vi "nanocal -- nuclear schottky fit V5.vi"() -> ()   [LabVIEW 2020] (continued)
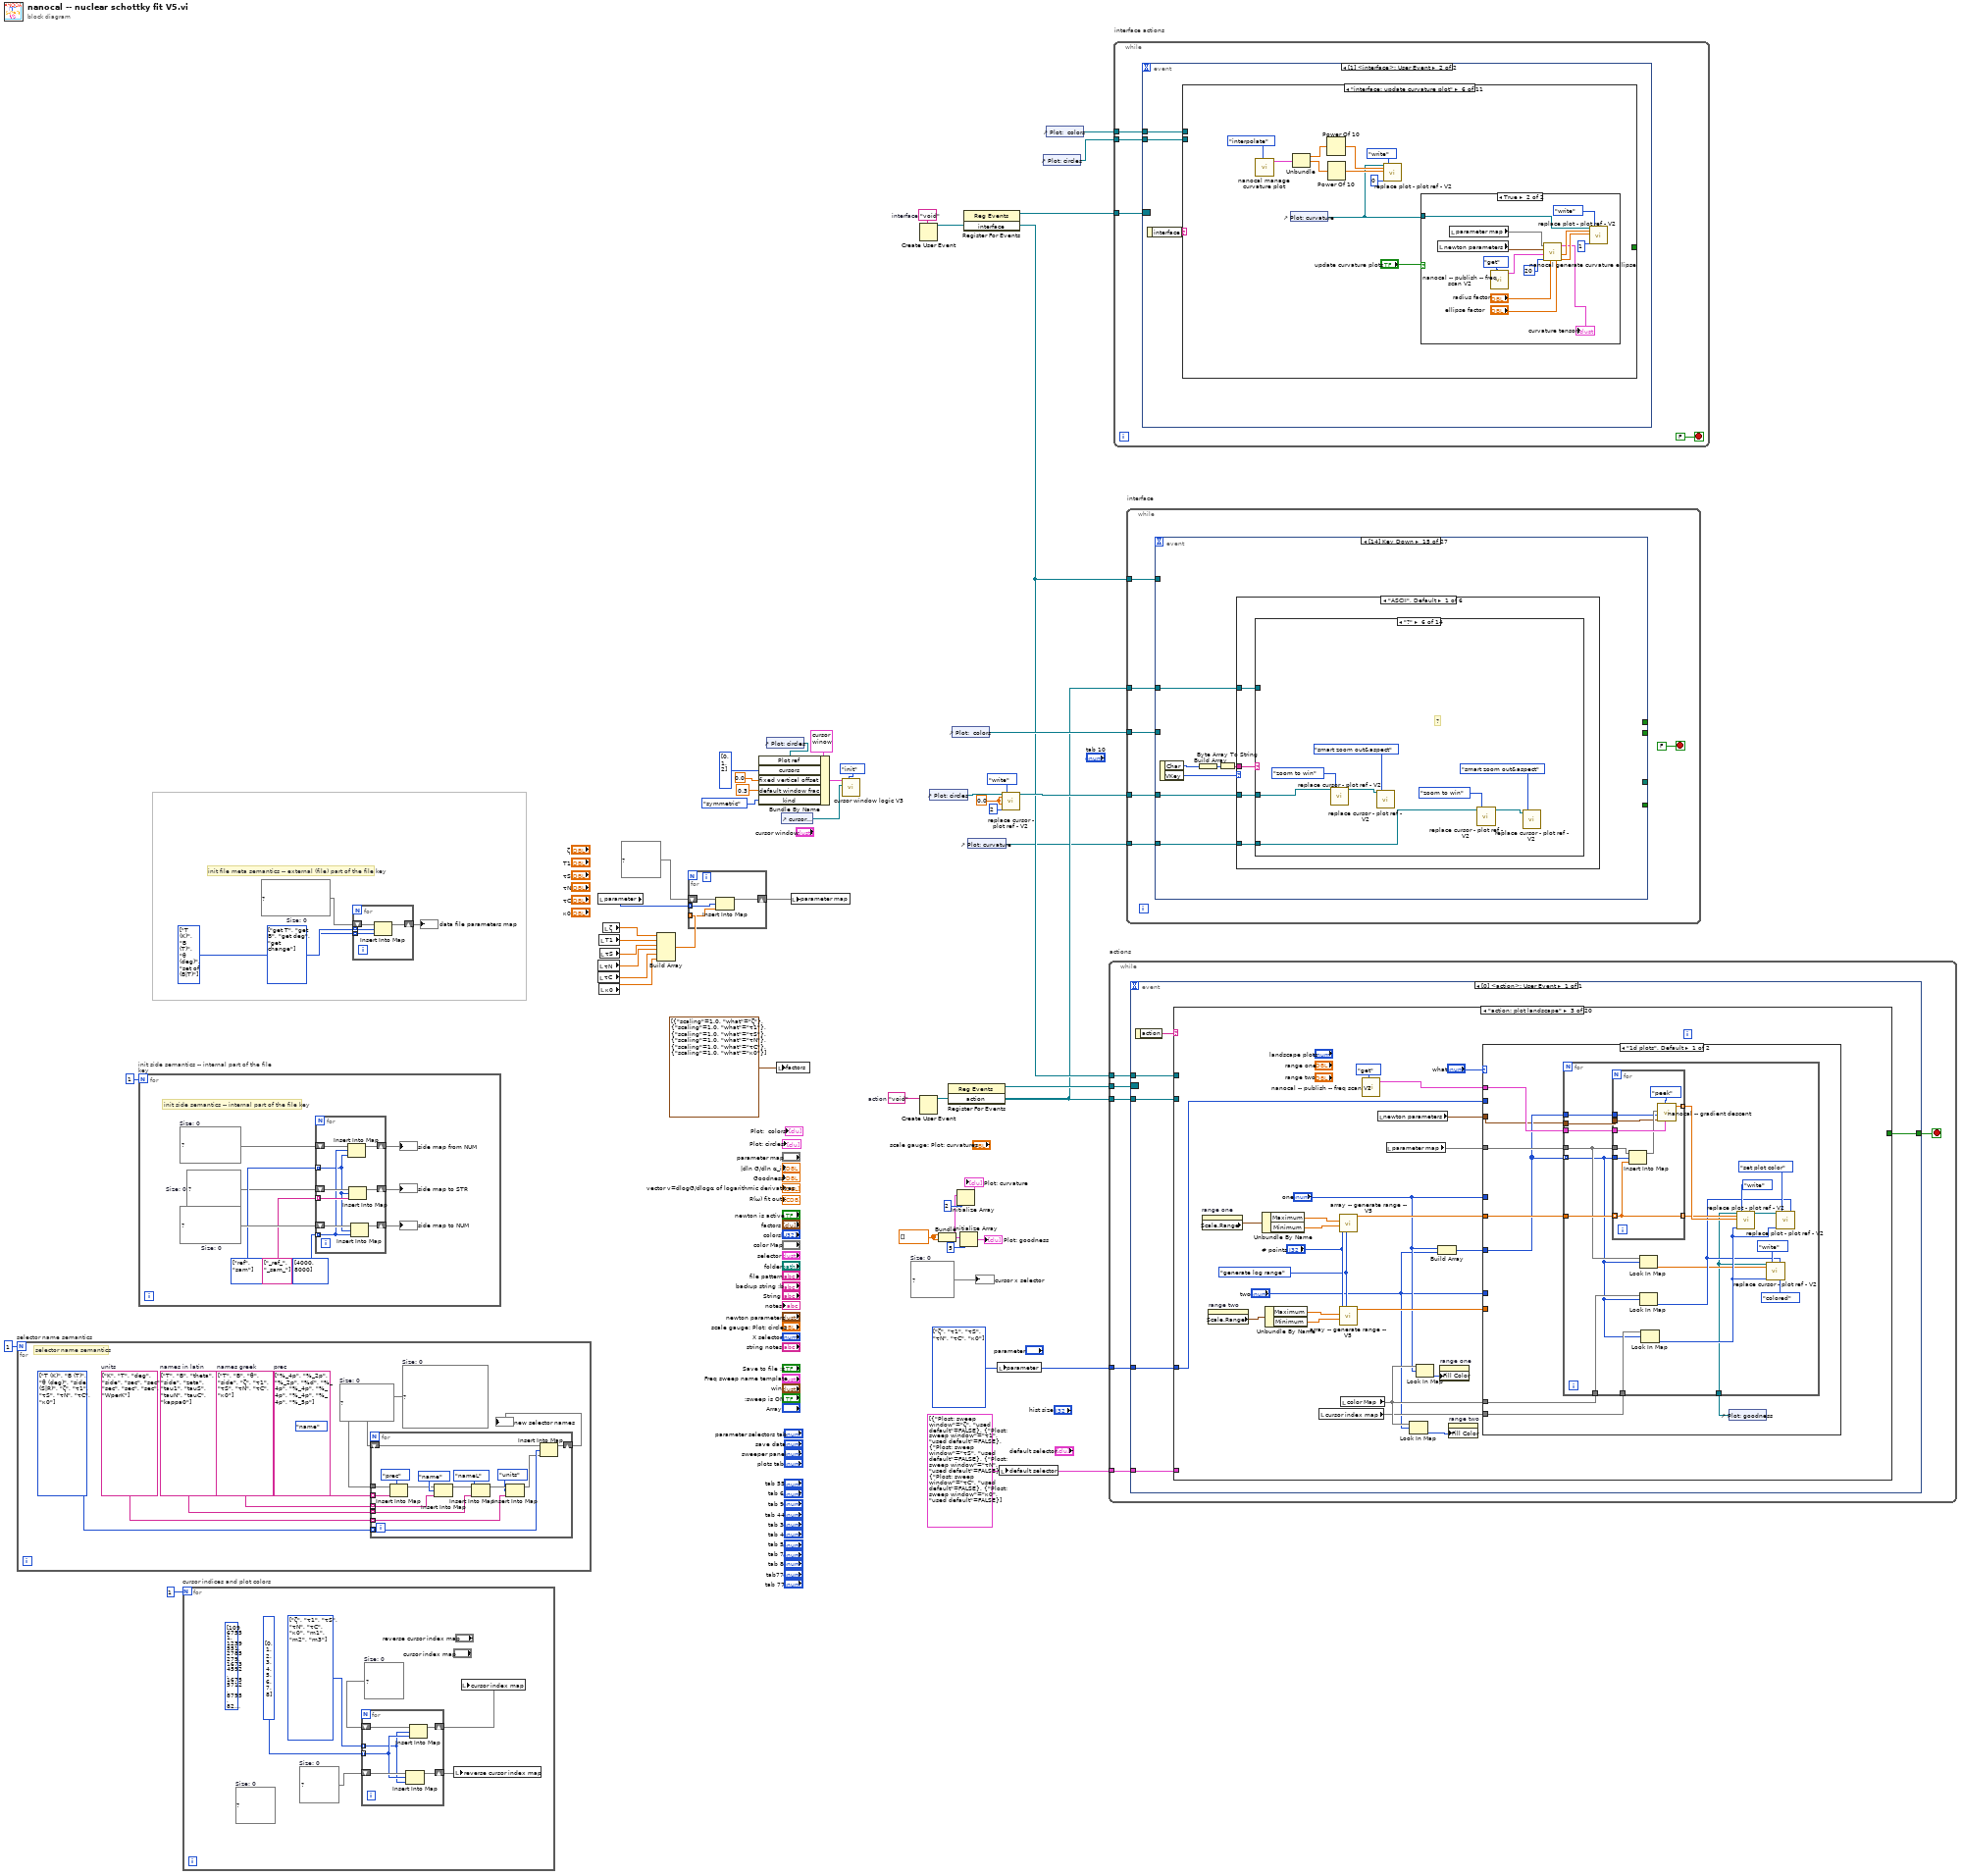
[diagram p0: block diagram]
diagram:
  w24 = T14 [{"Plost: sweep window"=enum."ζ", "used default"=FALSE}, {"Plost: sweep window"=enum."τ1", "used default"=FALSE}, {"Plost: sweep window"=enum."τS", "used default"=FALSE}, {"Plost: sweep window"=enum."τN", "used default"=FALSE}, {"Plost: sweep window"=enum."τC", "used default"=FALSE}, {"Plost: sweep window"=enum."κ0", "used default"=FALSE}] ("parameter 2")
  w25 = T12[] [enum."get T", enum."get B", enum."get deg", enum."get change"] items=["rewrite", "parse", "force pattern", "uniquenum", "get T", "get B", "get ind", "get deg", "get name", "get folder", "get extension", "get basename", "get side", "get change", "getID", "getIDStock"]
  w27 = map{T4, T12} {}  # Size: 0
  w26 = T4[] [enum."T (K)", enum."B (T)", enum."θ (deg)", enum."set of (B|T)"] items=["ζ", "τ1", "τS", "τN", "τC", "κ0", "m1", "m2", "m3", "T (K)", "B (T)", "θ (deg)", "side (S|R)", "set of (B|T)", "Re(offset)", "Im(offset)"]
  w31 = dbl[] []
  w20 = T4[] [enum."ζ", enum."τ1", enum."τS", enum."τN", enum."τC", enum."κ0"] items=["ζ", "τ1", "τS", "τN", "τC", "κ0", "m1", "m2", "m3", "T (K)", "B (T)", "θ (deg)", "side (S|R)", "set of (B|T)", "Re(offset)", "Im(offset)"]
  w34 = map{T4, dbl} {}  # Size: 0
  w35 = 0.0 ("new X")
  w48 = "void"  # interface
  w49 = "void"  # action
  # "init file meta semantics -- external (file) part of the file key"
  n1 = for "selector name semantics" {
    N: 1 -> [_]
    w51 = string[] ["%_4p", "%_2p", "%_2p", "%d", "%_4p", "%_4p", "%_4p", "%_4p", "%_4p", "%_5p"]  # prec
    w55 = map{T13, string} {}  # Size: 0
    (unwired) nameformattingitem."name" ("name formatting item")
    w53 = string[] ["K", "T", "deg", "side", "sec", "sec", "sec", "sec", "sec", "WperK"]  # units
    w56 = string[] ["T", "B", "theta", "side", "zeta", "tau1", "tauS", "tauN", "tauC", "kappa0"]  # names in latin
    w54 = string[] ["T", "B", "θ", "side", "ζ", "τ1", "τS", "τN", "τC", "κ0"]  # names greek
    w58 = map{T4, map{T13, string}} {}  # Size: 0
    w57 = T4[] [enum."T (K)", enum."B (T)", enum."θ (deg)", enum."side (S|R)", enum."ζ", enum."τ1", enum."τS", enum."τN", enum."τC", enum."κ0"] items=["ζ", "τ1", "τS", "τN", "τC", "κ0", "m1", "m2", "m3", "T (K)", "B (T)", "θ (deg)", "side (S|R)", "set of (B|T)", "Re(offset)", "Im(offset)"]
    # "selector name semantics"
    n2 = for {
      shift-right: [w73] -> w52
      shift-left: w58 -> [w74]
      tunnel: w56 -> [w64] mode=indexing
      tunnel: w57 -> [w72] mode=indexing
      tunnel: w55 -> [w62]
      tunnel: w54 -> [w63] mode=indexing
      tunnel: w53 -> [w65] mode=indexing
      tunnel: w51 -> [w61] mode=indexing
      n3 = Insert Into Map(map in=w62, key=nameformattingitem."prec", value=w61) -> (map out=w60:map{T13, string})  [unwired: 2 out]
      n4 = Insert Into Map(map in=w60, key=nameformattingitem."name", value=w63) -> (map out=w71:map{T13, string})  [unwired: 2 out]
      n5 = Insert Into Map(map in=w71, key=nameformattingitem."nameL" ("name formatting item"), value=w64) -> (map out=w70:map{T13, string})  [unwired: 2 out]
      n6 = Insert Into Map(map in=w70, key=nameformattingitem."units" ("name formatting item"), value=w65) -> (map out=w69:map{T13, string})  [unwired: 2 out]
      n7 = Insert Into Map(map in=w74, key=w72, value=w69) -> (map out=w73:map{T4, map{T13, string}})  [unwired: 2 out]
    }
    "new selector names" <- w52
  }
  n8 = for "init side semantics -- internal part of the file key" {
    N: 1 -> [_]
    w76 = map{i32, T11} {}  # Size: 0
    w78 = map{T11, string} {}  # Size: 0
    w79 = T11[] [enum."ref", enum."sam"] items=["sam", "ref"]
    w83 = map{T11, i32} {}  # Size: 0
    # "init side semantics -- internal part of the file key"
    n9 = for {
      shift-right: [w91] -> w80
      shift-left: w83 -> [w92]
      tunnel: string[] ["_ref_", "_sam_"] -> [w88] mode=indexing
      tunnel: i32[] [4000, 8000] -> [w85] mode=indexing
      tunnel: w79 -> [w84] mode=indexing
      shift-right: [w89] -> w77
      shift-left: w78 -> [w90]
      shift-right: [w86] -> w75
      shift-left: w76 -> [w87]
      n10 = Insert Into Map(map in=w87, key=w85, value=w84) -> (map out=w86:map{i32, T11})  [unwired: 2 out]
      n11 = Insert Into Map(map in=w90, key=w84, value=w88) -> (map out=w89:map{T11, string})  [unwired: 2 out]
      n12 = Insert Into Map(map in=w92, key=w84, value=w85) -> (map out=w91:map{T11, i32})  [unwired: 2 out]
    }
    "side map from NUM" <- w75
    "side map to STR" <- w77
    "side map to NUM" <- w80
  }
  n13 = for "cursor indices and plot colors" {
    N: 1 -> [_]
    (unwired) map{T4, i32} {}  # Size: 0
    w94 = map{i32, T4} {}  # Size: 0
    (unwired) u32[] [10967551, 1239551, 2785279, 16734592, 16755712, 8795, 8285330, 9272482, 9204890]
    w98 = map{T4, i32} {}  # Size: 0
    w95 = T4[] [enum."ζ", enum."τ1", enum."τS", enum."τN", enum."τC", enum."κ0", enum."m1", enum."m2", enum."m3"] items=["ζ", "τ1", "τS", "τN", "τC", "κ0", "m1", "m2", "m3", "T (K)", "B (T)", "θ (deg)", "side (S|R)", "set of (B|T)", "Re(offset)", "Im(offset)"]
    n14 = for {
      shift-right: [w103] -> w96
      shift-left: w98 -> [w104]
      tunnel: w95 -> [w99] mode=indexing
      tunnel: i32[] [0, 1, 2, 3, 4, 5, 6, 7, 8] -> [w100] mode=indexing
      shift-right: [w101] -> w93
      shift-left: w94 -> [w102]
      n15 = Insert Into Map(map in=w102, key=w100, value=w99) -> (map out=w101:map{i32, T4})  [unwired: 2 out]
      n16 = Insert Into Map(map in=w104, key=w99, value=w100) -> (map out=w103:map{T4, i32})  [unwired: 2 out]
    }
    n17 = local write "reverse cursor index map"(w93) -> ()
    n18 = local write "cursor index map"(w96) -> ()
  }
  n19 = for {
    shift-right: [w107] -> w28
    shift-left: w27 -> [w108]
    tunnel: w26 -> [w106] mode=indexing
    tunnel: w25 -> [w105] mode=indexing
    n20 = Insert Into Map(map in=w108, key=w106, value=w105) -> (map out=w107:map{T4, T12})  [unwired: 2 out]
  }
  "data file parameters map" <- w28
  n21 = local read "parameter"() -> (w18:T4[])
  n22 = local read "τN"() -> (w14:dbl)
  n23 = local read "τC"() -> (w15:dbl)
  n24 = local read "T1"() -> (w12:dbl)
  n25 = local read "κ0"() -> (w16:dbl)
  n26 = local read "τS"() -> (w13:dbl)
  n27 = local read "ζ"() -> (w11:dbl)
  n28 = Build Array(w11, w12, w13, w14, w15, w16) -> (w17:dbl[])
  n29 = for {
    shift-right: [w111] -> w19
    shift-left: map{T4, dbl} {} ("Map IN") -> [w112]
    tunnel: w18 -> [w110] mode=indexing
    tunnel: w17 -> [w109] mode=indexing
    n30 = Insert Into Map(map in=w112, key=w110, value=w109) -> (map out=w111:map{T4, dbl})  [unwired: 2 out]
  }
  n31 = control-ref of="Plot: circles"() -> (w40:refnum<vi>)
  n32 = Bundle By Name(cluster=T17 {"left"=0.0, "right "=0.0, "center"=0.0, "window"=0.0, "cursors"=[], "relative"=0, "absolute"=0, "fixed vertical offset"=0.0, "vertical offset"=0.0, "skew"=0.0, "default window frac"=0.0, "kind"=enum."symmetric", "skew.left"=0.0, "skew.right"=0.0, "Plot ref"=refnum, "wing order"=enum."forw"} ("cursor bracket: All, data window"), "Plot ref"=w40, "cursors"=i32[] [0, 1, 2], "fixed vertical offset"=0.0, "default window frac"=0.3 ("fixed vertical offset"), "kind"=enum16{"symmetric", "skewed", "fancy"}."symmetric") -> (w43:T17)
  n33 = local write "factors"(cluster{"scaling":dbl, "what":T4}[] [{"scaling"=1.0, "what"=enum."ζ"}, {"scaling"=1.0, "what"=enum."τ1"}, {"scaling"=1.0, "what"=enum."τS"}, {"scaling"=1.0, "what"=enum."τN"}, {"scaling"=1.0, "what"=enum."τC"}, {"scaling"=1.0, "what"=enum."κ0"}]) -> ()
  n34 = control-ref of="cursor window"() -> (w39:refnum<vi>)
  n35 = local write "parameter map"(w19) -> ()
  n36 = call "cursor window logic V3.vi"("cursor window action"=cursor_window_action."init", "cursor window in"=w39, "cursor window init"=w43) -> ()  [unwired: 7 in, 2 out]
  n37 = Create User Event(user event datatype=w48) -> (user event=w8:refnum<user-event>)  [unwired: 1 in, 1 out]
  n38 = Create User Event(user event datatype=w49) -> (user event=w7:refnum<user-event>)  [unwired: 1 in, 1 out]
  n39 = control-ref of="Plot: circles"() -> (w36:refnum<vi>)
  n40 = Bundle(w31, w31) -> (w3:cluster{dbl[], dbl[]})  [unwired: 1 in]
  n41 = register-events(w7) -> (reference out=w50:refnum<event-registration>)  [unwired: 2 in, 1 out]
  n42 = control-ref of="Plot:  colors"() -> (w33:refnum<vi>)
  n43 = Initialize Array(w3, 2 ("dimension size")) -> (→"Plot: curvature":cluster{dbl[], dbl[]}[])
  n44 = Initialize Array(w3, 5 ("dimension size")) -> (→"Plot: goodness":cluster{dbl[], dbl[]}[])
  n45 = register-events(w8) -> (reference out=w9:refnum<event-registration>)  [unwired: 2 in, 1 out]
  n46 = control-ref of="Plot: curvature"() -> (w1:refnum<vi>)
  n47 = local write "parameter"(w20) -> ()
  n48 = local write "default selector"(w24) -> ()
  n49 = call "replace cursor - plot ref - V2.vi"("Plot ref in"=w36, "new X"=w35, "new  Y"=w35, "cursor index"=2, "cursor action"=cursor_action."write") -> ()  [unwired: 11 in, 4 out]
  n50 = control-ref of="Plot: circles"() -> (w5:refnum<vi>)
  n51 = control-ref of="Plot:  colors"() -> (w6:refnum<vi>)
  n52 = while "actions" {
    tunnel: w50 -> [w118]
    tunnel: w7 -> [w117]
    tunnel: w8 -> [w115]
    tunnel: w20 -> [w114]
    tunnel: w24 -> [w113]
    stop <- w116 stop-if-true
    n53 = event shown="[0] <action>: User Event" {
      selector: w118 -> [_]
      dyn-events: _ -> [_]
      timeout: _ -> [_]
      tunnel: w117 -> [w123]
      tunnel: [w122] -> w116
      tunnel: w115 -> [w121]
      tunnel: w114 -> [w120]
      tunnel: w113 -> [w119]
      event User Event {
        n54 = event-data() -> ("action"=w124:string)  [unwired: 1 in]
        n55 = case shown="\"action: plot landscape\"" w124 {
          tunnel: w123 -> [w132 _ _ _ w328 w353 _ _ w546 _ w673 _ _ w777 w829 w910 _ w968 _ _]
          tunnel: [_ _ _ _ _ _ _ _ _ _ _ _ _ _ _ _ TRUE _ _ _] -> w122
          tunnel: w121 -> [w135 w139 _ w263 w322 _ _ _ _ _ _ _ w686 _ w819 _ _ _ _ _]
          tunnel: w120 -> [_ w146 w155 w262 _ _ w480 _ _ _ _ _ w687 _ w825 _ _ _ _ _]
          tunnel: w119 -> [_ _ _ _ _ _ _ _ _ _ _ _ _ _ _ _ _ _ _ _]
          frame "action: new sweep" {
            n56 = Generate User Event(user event=w135, event data cluster="interface: update plot colors cursors" ("event data")) -> (user event out=w136:refnum<user-event>)  [unwired: 2 in, 1 out]
            n57 = Generate User Event(user event=w136, event data cluster="interface: reset colors" ("event data")) -> ()  [unwired: 2 in, 2 out]
            n58 = Generate User Event(user event=w132, event data cluster="action: replot circles" ("event data")) -> ()  [unwired: 2 in, 2 out]
            n59 = call "nanocal -- publish -- freq scan V2.vi"("publisher action"=publisher_action."get") -> ("z out (V)"=w131:cdb[])  [unwired: 7 in, 3 out]
            n60 = control-ref of="Plot: circles"() -> (w126:refnum<vi>)
            n61 = Complex To Re/Im(x + iy=w131) -> (x=w129:dbl[], y=w130:dbl[])
            n62 = call "replace plot - plot ref - V2.vi"("Plot ref in"=w126, "Array X IN"=w129, "Array Y IN"=w130, "plot index"=enum16{"data R(ω)", "fit R(ω)"}."data R(ω)" ("Plost: sweep window"), "cursor action"=cursor_action."write") -> ()  [unwired: 11 in, 4 out]
          }
          frame "action: replot circles" {
            n63 = local read "newton parameters"() -> (w147:T5)
            n64 = local read "parameter map"() -> (w141:map{T4, dbl})
            n65 = call "nanocal -- publish -- freq scan V2.vi"("publisher action"=publisher_action."get") -> ("data"=w145:T32)  [unwired: 7 in, 3 out]
            n66 = call "nanocal -- gradient descent.vi"("data"=w145, "action"=nanocal_--_gradient_descent_--_action."peek", "newton pars"=w147, "parameter keys IN"=w146, "parameter Map IN"=w141) -> ("logarithmic derivatives OUT"=w142:dbl[], "R(ω) out"=w140:cdb[], "goodness OUT"=w144:dbl)  [unwired: 2 in, 2 out]
            n67 = flat-sequence {
              tunnel: w140 -> [w150]
              tunnel: w139 -> [w152]
              tunnel: "interface: update circle fit plot" ("event data") -> [w151]
              frame #0 {
                n68 = local write "R(ω) fit out"(w150) -> ()
              }
              frame #1 {
                n69 = Generate User Event(user event=w152, event data cluster=w151) -> ()  [unwired: 2 in, 2 out]
              }
            }
            n70 = local write "Goodness"(w144) -> ()
            n71 = Absolute Value(x=w142) -> (abs(x)=w143:dbl[])
            n72 = local write "|v_i| = | dlogG/dlogα_i | (log scale slider)"(w143) -> ()
            n73 = local write "vector v=dlogG/dlogα of logarithmic derivatives"(w142) -> ()
          }
          frame "action: plot landscape" {
            w166 = array_action."generate log range" ("action")
            n74 = property on="range one" class="Slide (strict)"() -> ("Scale.Range"=w175:T34)  [unwired: 2 in, 2 out]
            n75 = property on="range two" class="Slide (strict)"() -> ("Scale.Range"=w174:T34)  [unwired: 2 in, 2 out]
            n76 = Unbundle By Name(w175) -> ("Maximum"=w169:dbl, "Minimum"=w168:dbl)
            n77 = Unbundle By Name(w174) -> ("Maximum"=w171:dbl, "Minimum"=w170:dbl)
            n78 = local read "cursor index map"() -> (w161:map{T4, i32})
            n79 = call "array -- generate range -- V5.vi"("action"=w166, "ω points"="# points", "ω from"=w168, "ω to"=w169) -> ("ω out"=w167:dbl[])  [unwired: 7 in]
            n80 = call "array -- generate range -- V5.vi"("action"=w166, "ω points"="# points", "ω from"=w170, "ω to"=w171) -> ("ω out"=w172:dbl[])  [unwired: 7 in]
            n81 = local read "color Map"() -> (w162:map{T4, u32})
            n82 = call "nanocal -- publish -- freq scan V2.vi"("publisher action"=publisher_action."get") -> ("data"=w154:T32)  [unwired: 7 in, 3 out]
            n83 = local read "newton parameters"() -> (w156:T5)
            n84 = local read "parameter map"() -> (w153:map{T4, dbl})
            n85 = Look In Map(map=w162, key="two") -> (value=w164:u32)  [unwired: 1 in, 1 out]
            n86 = Look In Map(map=w162, key="one") -> (value=w163:u32)  [unwired: 1 in, 1 out]
            n87 = Build Array("one", "two") -> (w160:T4[])
            n88 = property on="range one" class="Slide (strict)"("Fill Color"=w163) -> ()  [unwired: 2 in, 2 out]
            n89 = property on="range two" class="Slide (strict)"("Fill Color"=w164) -> ()  [unwired: 2 in, 2 out]
            n90 = case shown="\"1d plots\", Default" "what" {
              tunnel: w153 -> [w183 w223]
              tunnel: "one" -> [_ w222]
              tunnel: w172 -> [_ w221]
              tunnel: w167 -> [w182 w220]
              tunnel: "two" -> [_ w219]
              tunnel: w162 -> [w181 _]
              tunnel: w161 -> [w180 _]
              tunnel: w160 -> [w177 _]
              tunnel: w154 -> [w178 w214]
              tunnel: w156 -> [w176 w212]
              tunnel: w155 -> [_ w213]
              frame "1d plots", Default {
                n91 = control-ref of="Plot: goodness"() -> (w179:refnum<vi>)
                n92 = for {
                  tunnel: w183 -> [w190]
                  tunnel: w182 -> [w199]
                  tunnel: w177 -> [w189] mode=indexing
                  tunnel: w181 -> [w196]
                  tunnel: w180 -> [w195]
                  tunnel: w179 -> [w187]
                  tunnel: w178 -> [w186]
                  tunnel: w177 -> [w185]
                  tunnel: w176 -> [w184]
                  n93 = for {
                    tunnel: w199 -> [w203] mode=indexing
                    tunnel: [w204] -> w201 mode=indexing
                    tunnel: [w203] -> w200 mode=indexing
                    tunnel: w190 -> [w210]
                    tunnel: w189 -> [w211]
                    tunnel: w186 -> [w209]
                    tunnel: w185 -> [w206]
                    tunnel: w184 -> [w205]
                    n94 = Insert Into Map(map in=w210, key=w211, value=w203) -> (map out=w208:map{T4, dbl})  [unwired: 2 out]
                    n95 = call "nanocal -- gradient descent.vi"("data"=w209, "action"=nanocal_--_gradient_descent_--_action."peek", "newton pars"=w205, "parameter keys IN"=w206, "parameter Map IN"=w208) -> ("goodness OUT"=w204:dbl)  [unwired: 2 in, 4 out]
                  }
                  n96 = Look In Map(map=w190, key=w189) -> (value=w188:dbl)  [unwired: 1 in, 1 out]
                  n97 = Look In Map(map=w196, key=w189) -> (value=w191:u32)  [unwired: 1 in, 1 out]
                  n98 = Look In Map(map=w195, key=w189) -> (value=w193:i32)  [unwired: 1 in, 1 out]
                  n99 = call "replace plot - plot ref - V2.vi"("Plot ref in"=w187, "Array X IN"=w200, "Array Y IN"=w201, "plot index"=w193, "cursor action"=cursor_action."write") -> ("Plot ref out"=w198:refnum<vi>)  [unwired: 11 in, 3 out]
                  n100 = call "replace cursor - plot ref - V2.vi"("Plot ref in"=w187, "new X"=w188, "cursor index"=w193, "cursor action"=cursor_action."write", "Color Box"=w191, "cursor state"=cursor_sate."colored") -> ()  [unwired: 10 in, 4 out]
                  n101 = call "replace plot - plot ref - V2.vi"("Plot ref in"=w198, "plot index"=w193, "cursor action"=cursor_action."set plot color", "Color Box"=w191) -> ()  [unwired: 12 in, 4 out]
                }
              }
              frame "2d plots " {
                n102 = for {
                  tunnel: w223 -> [w233]
                  tunnel: w222 -> [w232]
                  tunnel: w221 -> [w231] mode=indexing
                  tunnel: w220 -> [w230]
                  tunnel: w219 -> [w229]
                  shift-right: [w227] -> w216
                  shift-left: "{ " -> [w228]
                  tunnel: w214 -> [w226]
                  tunnel: w213 -> [w225]
                  tunnel: w212 -> [w224]
                  n103 = for {
                    tunnel: w230 -> [w241] mode=indexing
                    tunnel: w231 -> [w240]
                    tunnel: w233 -> [w254]
                    tunnel: w232 -> [w255]
                    tunnel: w229 -> [w253]
                    shift-right: [w250] -> w227
                    shift-left: w228 -> [w251]
                    tunnel: w226 -> [w238]
                    tunnel: w225 -> [w235]
                    tunnel: w224 -> [w234]
                    w244 = " ,     "
                    w249 = i16 12 ("precision (6)")
                    n104 = Insert Into Map(map in=w254, key=w255, value=w241) -> (map out=w252:map{T4, dbl})  [unwired: 2 out]
                    n105 = Number To Fractional String(number=w241, precision (6)=w249) -> (F-format string=w248:string)  [unwired: 2 in]
                    n106 = Number To Fractional String(number=w240, precision (6)=w249) -> (F-format string=w247:string)  [unwired: 2 in]
                    n107 = Insert Into Map(map in=w252, key=w253, value=w240) -> (map out=w239:map{T4, dbl})  [unwired: 2 out]
                    n108 = call "nanocal -- gradient descent.vi"("data"=w238, "action"=nanocal_--_gradient_descent_--_action."peek", "newton pars"=w234, "parameter keys IN"=w235, "parameter Map IN"=w239) -> ("goodness OUT"=w236:dbl)  [unwired: 2 in, 4 out]
                    n109 = Number To Fractional String(number=w236, precision (6)=w249) -> (F-format string=w246:string)  [unwired: 2 in]
                    n110 = Concatenate Strings(w251, "{    ", w248, w244, w247, w244, w246, " } , ", "\r") -> (w250:string)
                  }
                }
                n111 = Concatenate Strings(w216, " }   ") -> (→"2dplots":string)
              }
            }
          }
          frame "action: gradient step" {
            n112 = local read "hist size"() -> (w256:i32)
            n113 = local write "newton is active"(TRUE ("newton is active")) -> ()
            n114 = call "nanocal -- publish -- freq scan V2.vi"("publisher action"=publisher_action."get") -> ("data"=w264:T32)  [unwired: 7 in, 3 out]
            n115 = call "nanocal manage curvature plot.vi"("hist size"=w256, "aggregator action"=agregator_--_action."empty!") -> ("arrays OUT"=w257:T35)  [unwired: 6 in, 3 out]
            n116 = call "nanocal -- gradient descent.vi"("data"=w264, "action"=nanocal_--_gradient_descent_--_action."init") -> ("goodness OUT"=w266:dbl)  [unwired: 5 in, 4 out]
            n117 = while {
              tunnel: w266 -> [_]
              tunnel: w262 -> [w296]
              tunnel: w263 -> [w286]
              tunnel: [w281] -> w260
              tunnel: w257 -> [_]
              i -> [w282]
              stop <- w281 continue-if-true
              n118 = local read "newton is active"() -> (w297:bool)
              n119 = local read "factors"() -> (w300:cluster{"scaling":dbl, "what":T4}[])
              n120 = Quotient & Remainder(x=w282, y="update rate") -> (x-y*floor(x/y)=w285:i32)  [unwired: 1 out]
              n121 = local read "newton parameters"() -> (w295:T5)
              n122 = Less?(x=w282, y="total # steps") -> (x < y?=w283:bool)
              n123 = for {
                shift-right: [w320] -> w289
                shift-left: map{T4, dbl} {} ("Map IN") -> [w321]
                tunnel: w300 -> [w319] mode=indexing
                n124 = Unbundle(w319) -> ("scaling"=w317:dbl, "what"=w318:T4)
                n125 = Insert Into Map(map in=w321, key=w318, value=w317) -> (map out=w320:map{T4, dbl})  [unwired: 2 out]
              }
              n126 = local read "parameter map"() -> (w290:map{T4, dbl})
              n127 = And(x=w283, y=w297) -> (x .and. y?=w281:bool)
              n128 = case shown="0" w285 {
                tunnel: w286 -> [_ w304]
                frame 1, Default {
                }
                frame 0 {
                  n129 = Generate User Event(user event=w304, event data cluster="interface: update list from parameter map" ("event data")) -> (user event out=w303:refnum<user-event>)  [unwired: 2 in, 1 out]
                  n130 = Generate User Event(user event=w303, event data cluster="interface: update plot colors cursors" ("event data")) -> (user event out=w307:refnum<user-event>)  [unwired: 2 in, 1 out]
                  n131 = Generate User Event(user event=w307, event data cluster="interface: update circle fit plot" ("event data")) -> (user event out=w302:refnum<user-event>)  [unwired: 2 in, 1 out]
                  n132 = Generate User Event(user event=w302, event data cluster="interface: update curvature plot" ("event data")) -> ()  [unwired: 2 in, 2 out]
                }
              }
              n133 = call "nanocal -- gradient descent.vi"("# steps"="# plot steps", "action"=nanocal_--_gradient_descent_--_action."step", "newton pars"=w295, "parameter keys IN"=w296, "parameter Map IN"=w290, "factors Map IN"=w289) -> ("logarithmic derivatives OUT"=w291:dbl[], "step factors OUT"=w298:map{T4, dbl}, "R(ω) out"=w288:cdb[], "goodness OUT"=w276:dbl, "oscillations"=→"Plot: oscillations":cluster{"Array":i32[], "Array":dbl[]})  [unwired: 1 in]
              n134 = Logarithm Base 10(1:w276) -> (0:w275:dbl)
              n135 = local read "hist size"() -> (w268:i32)
              n136 = for {
                tunnel: w296 -> [w309] mode=indexing
                shift-right: [w313] -> _
                shift-left: w298 -> [w313]
                shift-right: [w311] -> w279
                shift-left: w290 -> [w312]
                n137 = Look In Map(map=w313, key=w309) -> (value=w310:dbl)  [unwired: 1 in, 1 out]
                n138 = in-place {
                  in-place-border: w310 -> [w315]
                  n139 = in-place-map #1(w312, w309) -> (w316:dbl)  [unwired: 1 in, 1 out]
                  n140 = Multiply(x=w315, y=w316) -> (x*y=w314:dbl)
                  n141 = in-place-map #1(w314) -> (w311:map{T4, dbl})  [unwired: 1 in, 2 out]
                }
              }
              n142 = Look In Map(map=w279, key=3-lorentzian-parameters."τ1") -> (value=w271:dbl)  [unwired: 1 in, 1 out]
              n143 = Look In Map(map=w279, key=3-lorentzian-parameters."τS") -> (value=w272:dbl)  [unwired: 1 in, 1 out]
              n144 = Logarithm Base 10(1:w271) -> (0:w274:dbl)
              n145 = Logarithm Base 10(1:w272) -> (0:w273:dbl)
              n146 = Bundle(w274, w273, w275) -> (w269:cluster{dbl, dbl, dbl})  [unwired: 1 in]
              n147 = call "nanocal manage curvature plot.vi"("hist size"=w268, "aggregator action"=agregator_--_action."append", "xyz IN"=w269) -> ()  [unwired: 5 in, 4 out]
              n148 = Absolute Value(x=w291) -> (abs(x)=→"|v_i| = | dlogG/dlogα_i | (log scale slider)":dbl[])
              n149 = local write "Goodness"(w276) -> ()
              n150 = local write "R(ω) fit out"(w288) -> ()
              n151 = local write "vector v=dlogG/dlogα of logarithmic derivatives"(w291) -> ()
              n152 = local write "parameter map"(w279) -> ()
              "current step ind" <- w282
            }
            n153 = local write "newton is active"(w260) -> ()
            "current plot ind" <- 0 ("plot ind")
          }
          frame "action: parse string" {
            n154 = local read "String"() -> (w330:string)
            n155 = Generate User Event(user event=w322, event data cluster="interface: update list from parameter map" ("event data")) -> ()  [unwired: 2 in, 2 out]
            n156 = call "string parse mathematica assosiated array.vi"("action"=mathematica_string_map_action."parse string" ("derivative"), "String in"=w330) -> ("Map OUT"=w324:map{T4, dbl})  [unwired: 8 in, 1 out]
            n157 = Generate User Event ("action User Event")(user event=w328, event data cluster="action: update state of selectors" ("event data")) -> (user event out=w325:refnum<user-event>)  [unwired: 2 in, 1 out]
            n158 = Generate User Event ("action User Event")(user event=w325, event data cluster="action: replot colors" ("event data")) -> ()  [unwired: 2 in, 2 out]
            n159 = local write "parameter map"(w324) -> ()
          }
          frame "action: read mathematica string" {
            w340 = map{string, path} {}  # Size: 0
            w355 = map{T4, dbl} {}  # Size: 0
            w352 = set{dbl} {}  # Size: 0
            w356 = map{string, map{T4, dbl}} {}  # Size: 0
            w346 = map{string, string} {}  # Size: 0
            n160 = local read "data file parameters map"() -> (w349:map{T4, T12})
            n161 = local read "file pattern"() -> (w343:string)
            n162 = local read "folder"() -> (w344:path)
            n163 = local read "side map to NUM"() -> (w347:map{T11, i32})
            n164 = local read "side map to STR"() -> (w348:map{T11, string})
            n165 = Generate User Event(user event=w353, event data cluster="action: update enums" ("event data")) -> ()  [unwired: 2 in, 2 out]
            n166 = call <vilib>:"Recursive File List.vi"("pattern"=w343, "Continue Recursing on Error? (F)"=TRUE, "Folder Path"=w344) -> ("All Files in Dir"=w341:path[])  [unwired: 4 in, 4 out]
            n167 = call "string parse mathematica list assosiated array -- V2.vi"("action"=3-lorentzian-heat-response_action."parse string" ("derivative"), "string IN"="string IN") -> ("Map OUT"=w357:map{string, map{T4, dbl}})  [unwired: 8 in, 1 out]
            n168 = for {
              tunnel: w341 -> [w365] mode=indexing
              shift-right: [w379] -> w331
              shift-left: w357 -> [w389]
              shift-right: [w376] -> w351
              shift-left: w346 -> [w388]
              shift-right: [w375] -> w350
              shift-left: w356 -> [w384]
              shift-right: [w386] -> w335
              shift-left: w352 -> [w378]
              shift-right: [w377] -> w334
              shift-left: w352 -> [w387]
              tunnel: w355 -> [w382]
              shift-right: [w372] -> w333
              shift-left: w352 -> [w385]
              shift-right: [w374] -> w336
              shift-left: w352 -> [w383]
              tunnel: w349 -> [w381]
              shift-right: [w373] -> w338
              shift-left: w352 -> [w380]
              tunnel: w347 -> [w370]
              tunnel: w348 -> [w369]
              shift-right: [w366] -> w345
              shift-left: w340 -> [w367]
              w368 = T11[] [enum."sam", enum."ref"] items=["sam", "ref"]
              n169 = Strip Path(path=w365) -> (name=w364:string)  [unwired: 1 out]
              n170 = call "filename-manage.vi"("filename-action"=filename-action."getIDStock", "file name IN"=w364) -> ("string OUT"=w371:string)  [unwired: 7 in, 2 out]
              n171 = for {
                tunnel: w381 -> [w415]
                tunnel: w364 -> [w392]
                tunnel: w371 -> [w404]
                shift-right: [w413] -> w379
                shift-left: w389 -> [w424]
                shift-right: [w419] -> w386
                shift-left: w378 -> [w412]
                shift-right: [w411] -> w377
                shift-left: w387 -> [w420]
                shift-right: [w405] -> w372
                shift-left: w385 -> [w418]
                shift-right: [w406] -> w374
                shift-left: w383 -> [w416]
                shift-right: [w407] -> w373
                shift-left: w380 -> [w414]
                shift-right: [w408] -> w375
                shift-left: w384 -> [w417]
                shift-right: [w409] -> w376
                shift-left: w388 -> [w423]
                tunnel: w370 -> [w397]
                tunnel: w382 -> [w402]
                tunnel: w369 -> [w399]
                tunnel: w368 -> [w396] mode=indexing
                shift-right: [w393] -> w366
                shift-left: w367 -> [w394]
                tunnel: w365 -> [w391]
                # "internal key"
                n172 = Look In Map(map=w399, key=w396) -> (value=w398:string)  [unwired: 1 in, 1 out]
                n173 = Look In Map(map=w397, key=w396) -> (value=w395:i32)  [unwired: 1 in, 1 out]
                n174 = Concatenate Strings(w404, w398) -> (w403:string)
                n175 = Insert Into Map(map in=w402, key=3-lorentzian-parameters."side (S|R)", value=w395) -> (map out=w401:map{T4, dbl})  [unwired: 2 out]
                n176 = for {
                  shift-right: [w430] -> w410
                  shift-left: w401 -> [w431]
                  tunnel: w415 -> [w429] mode=indexing
                  tunnel: w392 -> [w427]
                  n177 = Unbundle(w429) -> ("key"=w428:T4, "filename-action"=w426:T12)
                  n178 = call "filename-manage.vi"("filename-action"=w426, "file name IN"=w427) -> ("number OUT"=w425:dbl)  [unwired: 7 in, 2 out]
                  n179 = Insert Into Map(map in=w431, key=w428, value=w425) -> (map out=w430:map{T4, dbl})  [unwired: 2 out]
                }
                n180 = in-place {
                  in-place-border: [w473] -> w422
                  in-place-border: w410 -> [w472]
                  n181 = in-place-map #2(w424, w403) -> (w471:map{T4, dbl}, w473:bool)  [unwired: 1 in]
                  n182 = for {
                    tunnel: w472 -> [w479] mode=indexing
                    shift-right: [w477] -> w470
                    shift-left: w471 -> [w478]
                    n183 = Unbundle(w479) -> ("key"=w476:T4, "number OUT"=w475:dbl)
                    n184 = Insert Into Map(map in=w478, key=w476, value=w475) -> (map out=w477:map{T4, dbl})  [unwired: 2 out]
                  }
                  n185 = in-place-map #2(w470, LVMapReplaceAction."Modify Entry only if found" ("action")) -> (w413:map{string, map{T4, dbl}})  [unwired: 2 out]
                }
                n186 = Not(x=w422) -> (.not. x?=w421:bool)
                n187 = case shown="True" w421 {
                  tunnel: w423 -> [w439 w469]
                  tunnel: [w439 w468] -> w409
                  tunnel: w392 -> [_ w467]
                  tunnel: w403 -> [_ w441]
                  tunnel: w420 -> [w437 w466]
                  tunnel: [w437 w465] -> w411
                  tunnel: w412 -> [w438 w464]
                  tunnel: [w438 w463] -> w419
                  tunnel: [w435 w462] -> w405
                  tunnel: w418 -> [w435 w461]
                  tunnel: w410 -> [_ w446]
                  tunnel: w417 -> [w436 w460]
                  tunnel: [w436 w459] -> w408
                  tunnel: [w434 w458] -> w406
                  tunnel: w416 -> [w434 w457]
                  tunnel: [w433 w448] -> w407
                  tunnel: w414 -> [w433 w447]
                  tunnel: w394 -> [w432 w443]
                  tunnel: [w432 w442] -> w393
                  tunnel: w391 -> [_ w440]
                  frame False {
                  }
                  frame True {
                    n188 = Look In Map(map=w446, key=3-lorentzian-parameters."set of (B|T)") -> (value=w449:dbl)  [unwired: 1 in, 1 out]
                    n189 = Look In Map(map=w446, key=3-lorentzian-parameters."side (S|R)") -> (value=w455:dbl)  [unwired: 1 in, 1 out]
                    n190 = Look In Map(map=w446, key=3-lorentzian-parameters."T (K)") -> (value=w453:dbl)  [unwired: 1 in, 1 out]
                    n191 = Look In Map(map=w446, key=3-lorentzian-parameters."B (T)") -> (value=w445:dbl)  [unwired: 1 in, 1 out]
                    n192 = Look In Map(map=w446, key=3-lorentzian-parameters."θ (deg)") -> (value=w444:dbl)  [unwired: 1 in, 1 out]
                    n193 = Insert Into Set(10:w449, 11:w447) -> (3:w448:set{dbl})  [unwired: 1 out]
                    n194 = Insert Into Set(10:w455, 11:w457) -> (3:w458:set{dbl})  [unwired: 1 out]
                    n195 = Insert Into Set(10:w453, 11:w461) -> (3:w462:set{dbl})  [unwired: 1 out]
                    n196 = Insert Into Set(10:w445, 11:w466) -> (3:w465:set{dbl})  [unwired: 1 out]
                    n197 = Insert Into Set(10:w444, 11:w464) -> (3:w463:set{dbl})  [unwired: 1 out]
                    n198 = Insert Into Map(map in=w460, key=w441, value=w446) -> (map out=w459:map{string, map{T4, dbl}})  [unwired: 2 out]
                    n199 = Insert Into Map(map in=w469, key=w441, value=w467) -> (map out=w468:map{string, string})  [unwired: 2 out]
                    n200 = Insert Into Map(map in=w443, key=w441, value=w440) -> (map out=w442:map{string, path})  [unwired: 2 out]
                  }
                }
              }
            }
            "all short filenames" <- w351
            "temps&degs" <- w350
            "mathematica thing" <- w331
            "all full filenames" <- w345
            n201 = local read "selector"() -> (w339:T15)
            n202 = in-place {
              in-place-border: w338 -> [w363]
              in-place-border: w336 -> [w362]
              in-place-border: w335 -> [w359]
              in-place-border: w334 -> [w360]
              in-place-border: w333 -> [w361]
              n203 = in-place-cluster #3(w339) -> ()  [unwired: 5 out]
              n204 = in-place-cluster #3("lookup.all set of"=w363, "lookup.all sides"=w362, "lookup.all T's"=w361, "lookup.all B's"=w360, "lookup.all θ's"=w359) -> (w337:T15)
            }
            n205 = local write "selector"(w337) -> ()
          }
          frame "action: update default values" {
            w484 = map{T4, cluster{"ζ":dbl, "ζ":dbl}[]} {}  # Size: 0
            (unwired) map{string, map{T4, dbl}} {} ("Map OUT")
            w482 = map{T4, dbl[]} {}  # Size: 0
            n206 = call "string parse mathematica list assosiated array -- V2.vi"("action"=3-lorentzian-heat-response_action."parse string" ("derivative"), "string IN"="default values string") -> ("Map OUT"=w485:map{string, map{T4, dbl}})  [unwired: 8 in, 1 out]
            n207 = for {
              tunnel: w485 -> [w511] mode=indexing
              tunnel: w480 -> [w510]
              shift-right: [w508] -> w483
              shift-left: w484 -> [w507]
              n208 = Unbundle(w511) -> ("Map"=w509:map{T4, dbl})  [unwired: 1 out]
              n209 = for {
                tunnel: w510 -> [w519] mode=indexing
                tunnel: w509 -> [w518]
                shift-right: [w513] -> w508
                shift-left: w507 -> [w512]
                # "parameter"
                # "temperatures"
                n210 = Look In Map(map=w518, key=w519) -> (value=w515:dbl)  [unwired: 1 in, 1 out]
                n211 = Look In Map(map=w512, key=w519) -> (value=w521:cluster{"ζ":dbl, "ζ":dbl}[])  [unwired: 1 in, 1 out]
                n212 = Look In Map(map=w518, key=3-lorentzian-parameters."T (K)" ("Plost: sweep window")) -> (value=w516:dbl)  [unwired: 1 in, 1 out]
                n213 = Bundle("ζ"=w516, "ζ"=w515) -> (w514:cluster{"ζ":dbl, "ζ":dbl})  [unwired: 1 in]
                n214 = Build Array (concatenate)(w521, w514) -> (w520:cluster{"ζ":dbl, "ζ":dbl}[])
                n215 = Insert Into Map(map in=w512, key=w519, value=w520) -> (map out=w513:map{T4, cluster{"ζ":dbl, "ζ":dbl}[]})  [unwired: 2 out]
              }
            }
            n216 = for {
              tunnel: w483 -> [w500] mode=indexing
              shift-right: [w497] -> w481
              shift-left: w482 -> [w496]
              # "sorted temperastures"
              # "parameter"
              # "temperastures"
              n217 = Unbundle(w500) -> ("Plost: sweep window"=w494:T4, w499:cluster{"ζ":dbl, "ζ":dbl}[])
              n218 = for {
                tunnel: w499 -> [w506] mode=indexing
                tunnel: [w505] -> w498 mode=indexing
                tunnel: [w504] -> w491 mode=indexing
                n219 = Unbundle(w506) -> ("ζ"=w505:dbl, "ζ"=w504:dbl)
              }
              n220 = call "array - sorted inexes.vi"("x"=w498) -> ("index array"=w490:i32[], "sorted array"=w492:dbl[])  [unwired: 9 in]
              n221 = Insert Into Map(map in=w496, key=3-lorentzian-parameters."T (K)", value=w492) -> (map out=w495:map{T4, dbl[]})  [unwired: 2 out]
              n222 = for {
                tunnel: w491 -> [w503]
                tunnel: w490 -> [w502] mode=indexing
                tunnel: [w501] -> w489 mode=indexing
                n223 = Index Array(array=w503, index=w502) -> (element=w501:dbl)
              }
              n224 = Insert Into Map(map in=w495, key=w494, value=w489) -> (map out=w497:map{T4, dbl[]})  [unwired: 2 out]
            }
            n225 = disable-structure shown="Disabled" {
              frame Disabled {
                # "2 3 4 0 1"
                # "2 3 4 5 6"
                # "5 6 2 3 4"
                n226 = call "array - sorted inexes.vi"() -> ()  [unwired: 10 in, 2 out]
              }
              frame Enabled {
              }
            }
            n227 = call "nanocal -- defaut parameter manager -- V1.vi"("action"=nanocal_--_defaut_parameter_manager_action--_V1."update", "internal map"=w481) -> ()  [unwired: 9 in, 1 out]
          }
          frame "action: empty string from filelist" {
            n228 = local read "file pattern"() -> (w523:string)
            n229 = local read "folder"() -> (w524:path)
            n230 = call <vilib>:"Recursive File List.vi"("pattern"=w523, "Continue Recursing on Error? (F)"=TRUE, "Folder Path"=w524) -> ("All Files in Dir"=w522:path[])  [unwired: 4 in, 4 out]
            n231 = for {
              tunnel: [w529] -> w526 mode=concatenating
              tunnel: w522 -> [w534] mode=indexing
              w532 = T11[] [enum."ref", enum."sam"] items=["sam", "ref"]
              n232 = Strip Path(path=w534) -> (name=w533:string)  [unwired: 1 out]
              n233 = local read "side map to STR"() -> (w531:map{T11, string})
              n234 = call "filename-manage.vi"("filename-action"=filename-action."getIDStock", "file name IN"=w533) -> ("string OUT"=w530:string)  [unwired: 7 in, 2 out]
              n235 = for {
                tunnel: w532 -> [w539] mode=indexing
                tunnel: w531 -> [w540]
                tunnel: w530 -> [w538]
                tunnel: [w536] -> w529 mode=indexing
                n236 = Look In Map(map=w540, key=w539) -> (value=w537:string)  [unwired: 1 in, 1 out]
                n237 = Concatenate Strings(w538, w537) -> (w536:string)
              }
            }
            n238 = call "string parse mathematica list assosiated array -- V2.vi"("action"=3-lorentzian-heat-response_action."create emty string" ("derivative"), "array of IDs"=w526) -> ("string out"=w527:string)  [unwired: 8 in, 1 out]
            n239 = local write "string OUT"(w527) -> ()
          }
          frame "action: update enums" {
            w544 = map{string, string} {}  # Size: 0
            w550 = map{i32, string} {}  # Size: 0
            # "gives a key"
            n240 = local read "selector"() -> (w542:T15)
            n241 = local read "all short filenames"() -> (w545:map{string, string})
            n242 = in-place {
              w567 = map{i32, dbl} {}  # Size: 0
              w573 = map{i32, dbl} {}  # Size: 0
              w574 = map{i32, dbl} {}  # Size: 0
              w576 = map{i32, dbl} {}  # Size: 0
              w575 = map{i32, dbl} {}  # Size: 0
              n243 = in-place-cluster #4(w542) -> ("lookup.all set of"=w561:set{dbl}, "lookup.all sides"=w560:set{dbl}, "lookup.all T's"=w559:set{dbl}, "lookup.all θ's"=w558:set{dbl}, "lookup.all B's"=w557:set{dbl})  [unwired: 5 out]
              n244 = for {
                shift-right: [w580] -> w566
                shift-left: w567 -> [w581]
                tunnel: [w578] -> w568 mode=indexing
                tunnel: w561 -> [w577] mode=indexing
                i -> [w579]
                n245 = Number To Decimal String(number=w577) -> (decimal integer string=w578:string)  [unwired: 1 in]
                n246 = Insert Into Map(map in=w581, key=w579, value=w577) -> (map out=w580:map{i32, dbl})  [unwired: 2 out]
              }
              n247 = for {
                shift-right: [w591] -> w563
                shift-left: w574 -> [w592]
                tunnel: [w589] -> w570 mode=indexing
                tunnel: w559 -> [w588] mode=indexing
                i -> [w590]
                n248 = Number To Fractional String(number=w588, precision (6)=i16 3) -> (F-format string=w589:string)  [unwired: 2 in]
                n249 = Insert Into Map(map in=w592, key=w590, value=w588) -> (map out=w591:map{i32, dbl})  [unwired: 2 out]
              }
              n250 = property on="set (1T|2B)" class="Ring (strict)"("Strings []"=w568) -> ()  [unwired: 2 in, 2 out]
              n251 = property on="T (K)" class="Ring (strict)"("Strings []"=w570) -> ()  [unwired: 2 in, 2 out]
              n252 = for {
                shift-right: [w585] -> w565
                shift-left: w573 -> [w586]
                tunnel: [w583] -> w569 mode=indexing
                tunnel: w560 -> [w582] mode=indexing
                i -> [w584]
                n253 = Number To Decimal String(number=w582) -> (decimal integer string=w583:string)  [unwired: 1 in]
                n254 = Insert Into Map(map in=w586, key=w584, value=w582) -> (map out=w585:map{i32, dbl})  [unwired: 2 out]
              }
              n255 = property on="side (8S|4R)" class="Ring (strict)"("Strings []"=w569) -> ()  [unwired: 2 in, 2 out]
              n256 = for {
                shift-right: [w603] -> w562
                shift-left: w575 -> [w604]
                tunnel: [w601] -> w571 mode=indexing
                tunnel: w558 -> [w600] mode=indexing
                i -> [w602]
                n257 = Number To Fractional String(number=w600, precision (6)=i16 3) -> (F-format string=w601:string)  [unwired: 2 in]
                n258 = Insert Into Map(map in=w604, key=w602, value=w600) -> (map out=w603:map{i32, dbl})  [unwired: 2 out]
              }
              n259 = for {
                shift-right: [w597] -> w564
                shift-left: w576 -> [w598]
